vi "FTW-JSON-Duplicate.vi"(0 "JSON Object":refnum<class "FTW-JSON.lvclass">, 11 "error in":errorcluster) -> (4 "JSON Object out":refnum<class "FTW-JSON.lvclass">, 6 "Duplicated JSON Object":refnum<class "FTW-JSON.lvclass">, 15 "error out":errorcluster)   [LabVIEW 2013, in "FTW-JSON.lvclass"]
uses:
  FTW-JSON.lvclass
  FTW-JSON.lvclass/FTW-JSON.ctl
  error/FTW-ERR-ThrowGenericError.vi
  error/FTW-ERR-ThrowError.vi
  error/FTW-ERR-NoErrorConstant.vi
  error/FTW-ERR-CallChain.vi
  string/FTW-STR-ReplaceWhitespace.vi
panel:
  # "Inputs"
  # "Outputs"
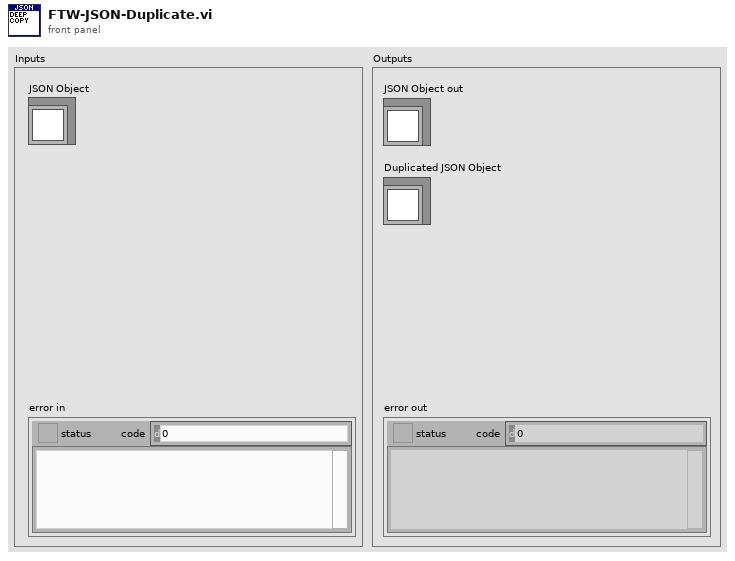
[diagram p1: front panel]
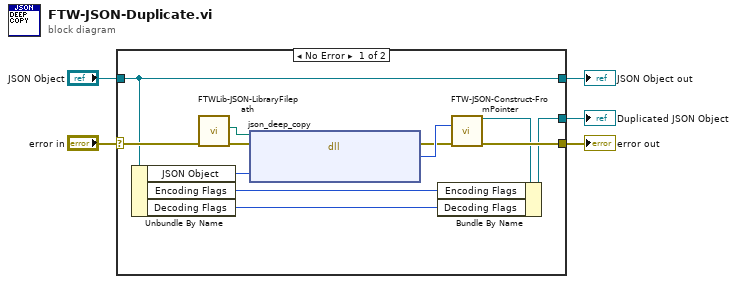
[diagram p0: block diagram]
diagram:
  n1 = case shown="No Error" "error in" {
    selector: "error in" -> [w17 w19]
    tunnel: [w10 w19] -> w5
    tunnel: "JSON Object" -> [w13 w18]
    tunnel: [w13 w18] -> w2
    tunnel: [w8 _] -> w1
    frame No Error {
      n2 = Unbundle By Name(w13) -> ("JSON Object"=w14:i64, "Encoding Flags"=w7:i64, "Decoding Flags"=w6:i64)
      n3 = call "FTWLib-JSON-LibraryFilepath.vi"("error in"=w17) -> ("error out"=w16:errorcluster, "JSON Library Filepath"=w15:path)  [unwired: 9 in]
      n4 = dll-call lib="?" fn="json_deep_copy"(path in=w15, error in=w16, "Original JSON Object Pointer"=w14) -> (error out=w11:errorcluster, "Duplicate JSON Object Pointer"=w12:i64)  [unwired: 2 in, 1 out]
      n5 = call "FTW-JSON-Construct-FromPointer.vi"("JSON Object Pointer"=w12, "error in"=w11) -> ("JSON Object"=w9:refnum<class "FTW-JSON.lvclass">, "error out"=w10:errorcluster)  [unwired: 12 in]
      n6 = Bundle By Name(cluster=w9, "Encoding Flags"=w7, "Decoding Flags"=w6) -> (w8:refnum<class "FTW-JSON.lvclass">)
    }
    frame Error {
    }
  }
  "error out" <- w5
  "Duplicated JSON Object" <- w1
  "JSON Object out" <- w2
